vi "MFL_Open_Queue.vi"(8 "error in (no error)":errorcluster caption="Fehler (Eingang, kein Fehler)") -> (0 "error out":errorcluster caption="Fehler (Ausgang)", 2 "queue out":refnum<queue>)   [LabVIEW 2019]
uses:
  Berta/15T-Control.ctl
  Global/Global Variables/Queues_global.vi
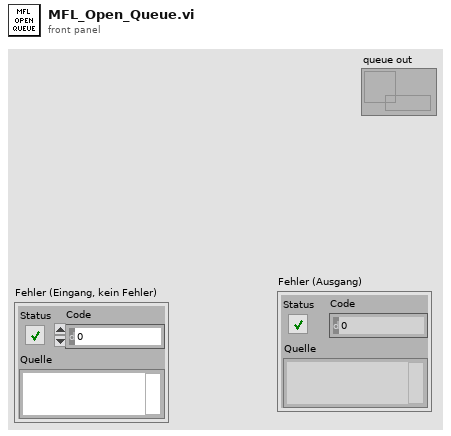
[diagram p1: front panel]
types:
  T1 = typedef "15T-Control.ctl" = cluster{"Setpoint (T)":dbl, "Rate (T/min)":dbl, "Go to zero":bool, "Go to Hold":bool, "Go to Set":bool, "Clamp":bool, "Switch Heater":bool}
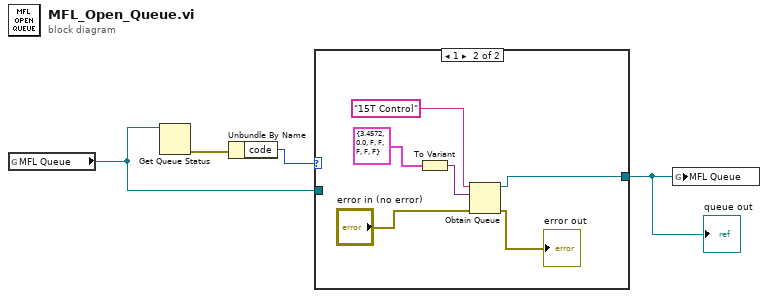
[diagram p0: block diagram]
diagram:
  n1 = global read "Queues_global.vi" "MFL Queue"() -> (w2:refnum<queue>)
  n2 = Get Queue Status(queue=w2) -> (error out=w4:errorcluster)  [unwired: 2 in, 7 out]
  n3 = Unbundle By Name(w4) -> ("code"=w3:i32)
  n4 = case shown="1" w3 {
    tunnel: w2 -> [w5 _]
    tunnel: [w5 w6] -> w1
    frame 0, Default {
    }
    frame 1 {
      n5 = To Variant(anything=T1 {"Setpoint (T)"=3.4572, "Rate (T/min)"=0.0, "Go to zero"=FALSE, "Go to Hold"=FALSE, "Go to Set"=FALSE, "Clamp"=FALSE, "Switch Heater"=FALSE} ("15T-Control")) -> (Variant=w8:variant)
      n6 = Obtain Queue(name (unnamed)="15T Control", element data type=w8, error in (no error)="error in (no error)") -> (queue out=w6:refnum<queue>, error out=→"error out":errorcluster)  [unwired: 2 in, 1 out]
    }
  }
  "queue out" <- w1
  n7 = global write "Queues_global.vi" "MFL Queue"(w1) -> ()
